vi "buildArrayTest.vi"() -> ()   [LabVIEW 2016]
uses:
  <vilib>/Analysis/Matrix/Datatypes/RealMatrix.ctl
  <vilib>/Analysis/Matrix/Numeric/Conversions/Array To Matrix - RA2.vi
  <vilib>/Analysis/Matrix/NI_Matrix.lvlib
panel:
  out "subarray":dbl[](array[numeric])=[5.0, 6.0]
  out "appended array 2":T1=[[-1.0, 1.0, 1.0], [-1.0, 1.0, 2.0], [-1.0, 1.0, 3.0], [-1.0, 1.0, 4.0], [-1.0, 1.0, 5.0], [1.0, -1.0, 6.0]]
  out "appended array":dbl[][](array[numeric])=[[-1.0, -1.0, -1.0, -1.0, -1.0, 1.0], [1.0, 1.0, 1.0, 1.0, 1.0, -1.0], [1.0, 2.0, 3.0, 4.0, 5.0, 6.0]]
  in  "Array 3":dbl[](array[numeric])=[1.0, 2.0, 3.0, 4.0, 5.0, 6.0]
  in  "Array 2":dbl[](array[numeric])=[1.0, 1.0, 1.0, 1.0, 1.0, -1.0]
  in  "Array":dbl[](array[numeric])=[-1.0, -1.0, -1.0, -1.0, -1.0, 1.0]
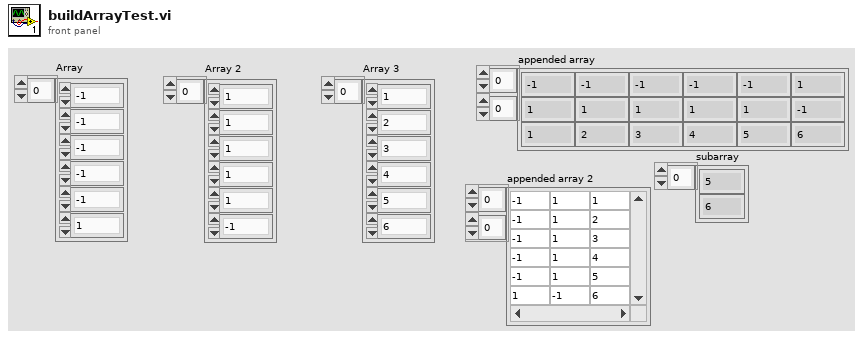
[diagram p1: front panel]
types:
  T1 = typedef "NI_Matrix.lvlib/RealMatrix.ctl" = dbl[][]
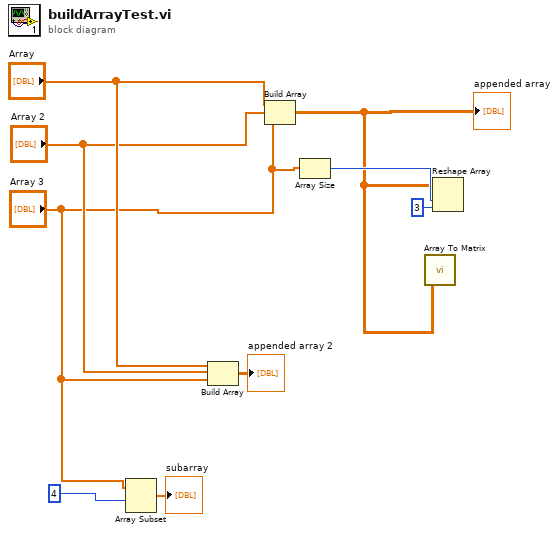
[diagram p0: block diagram]
diagram:
  n1 = Array Subset(array="Array 3", index=4) -> (→"subarray":dbl[])  [unwired: 1 in]
  n2 = Build Array("Array", "Array 2", "Array 3") -> (→"appended array 2":T1)
  n3 = Build Array("Array", "Array 2", "Array 3") -> (w7:dbl[][])
  "appended array" <- w7
  n4 = Array Size(array="Array 3") -> (size(s)=w9:i32)
  n5 = call-poly <vilib>:"Array To Matrix.vi"("Real 2D Array"=w7) -> ()  [unwired: 1 out]
  n6 = Reshape Array(w7, w9, 3 ("dimension size")) -> ()  [unwired: 1 out]
